vi "Get Keywords.vi"(8 "error in (no error)":errorcluster, 11 "Numeric Functions in":refnum<class "Numeric Functions.lvclass">) -> (0 "error out":errorcluster, 2 "Keywords":string[](array[string]), 3 "Numeric Functions out":refnum<class "Numeric Functions.lvclass">)   [LabVIEW 2019, in "Numeric Functions.lvclass"]
uses:
  Numeric Functions.lvclass
  functionsbase/functionbase.lvclass
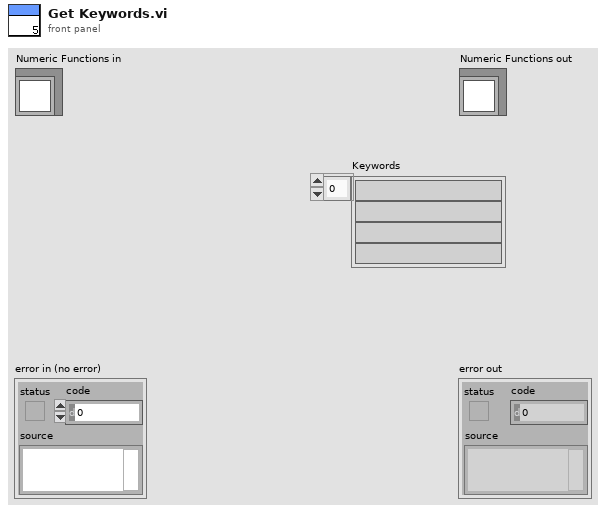
[diagram p1: front panel]
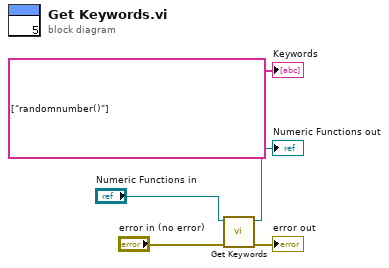
[diagram p0: block diagram]
diagram:
  n1 = call-parent "Get Keywords.vi"("error in (no error)"="error in (no error)", "functionbase in"="Numeric Functions in") -> ("error out"=→"error out":errorcluster, "functionbase out"=→"Numeric Functions out":refnum<class "Numeric Functions.lvclass">)  [unwired: 7 in, 1 out]
  "Keywords" <- string[] ["randomnumber()"] ("Keywords")
